vi "MultiScanDrift_v2.vi"() -> ()   [LabVIEW 2014]
uses:
  shared/CorrelImages (SubVI)Single.vi
  <userlib>/Nanonis Prog Interface V5/Nanonis Prog Interface.lvlib
panel:
  out "Direction: up/down (T=up)":bool
  in  "PLL ON/OFF":bool
  in  "ref bias":dbl=-0.0012 format="%#_6p"
  in  "ref setpoint":bool=TRUE
  in  "DC On":bool
  out "Y drift":i32
  out "X drift":i32
  out "DC active":bool
  in  "Drift correction Pixels":i32=256
  in  "Img Current":sgl=2.5e-11 format="%#_6p"
  in  "Img Bias (V) DC":sgl=0.02 format="%_2p"
  in  "Forward Speed":sgl=5e-10 format="%#_6p"
  in  "Backward Speed":sgl=8e-08 format="%#_6p"
  in  "Img Speed":sgl=3e-08 format="%#_6p"
  in  "Channel index (0-23)":u8(ring) items=["Current"=0, "Z (m)"=14]
  in  "Settling time (s)":dbl=0.7 format="%#_6p"
  in  "img bias":bool=TRUE
  in  "img bias":dbl=-0.0012 format="%#_6p"
  in  "img delay (s)":u32=1
  out "tipLift":dbl=1e-10 format="%#_6p"
  in  "TipLiftList":i32(listbox)
  in  "Const Height":bool=TRUE
  in  "CurrentList":i32(listbox)
  in  "BiasList":i32(listbox)
  out "Current":dbl=2.5e-11 format="%#_6p"
  out "Bias":dbl=0.02 format="%#_6p"
  # "Turn continuous scan off\n zero tiplift is '0'"
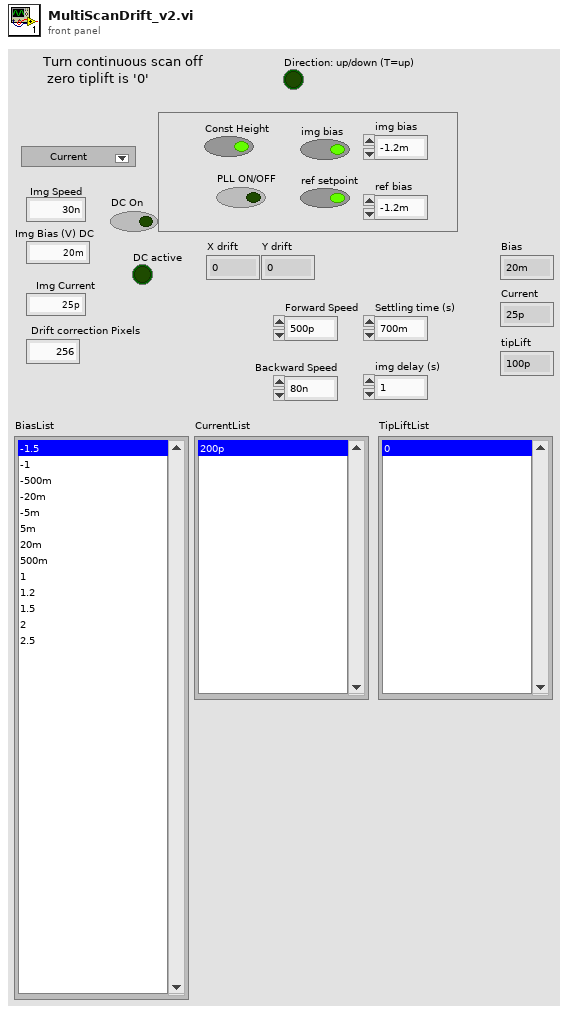
[diagram p1: front panel]
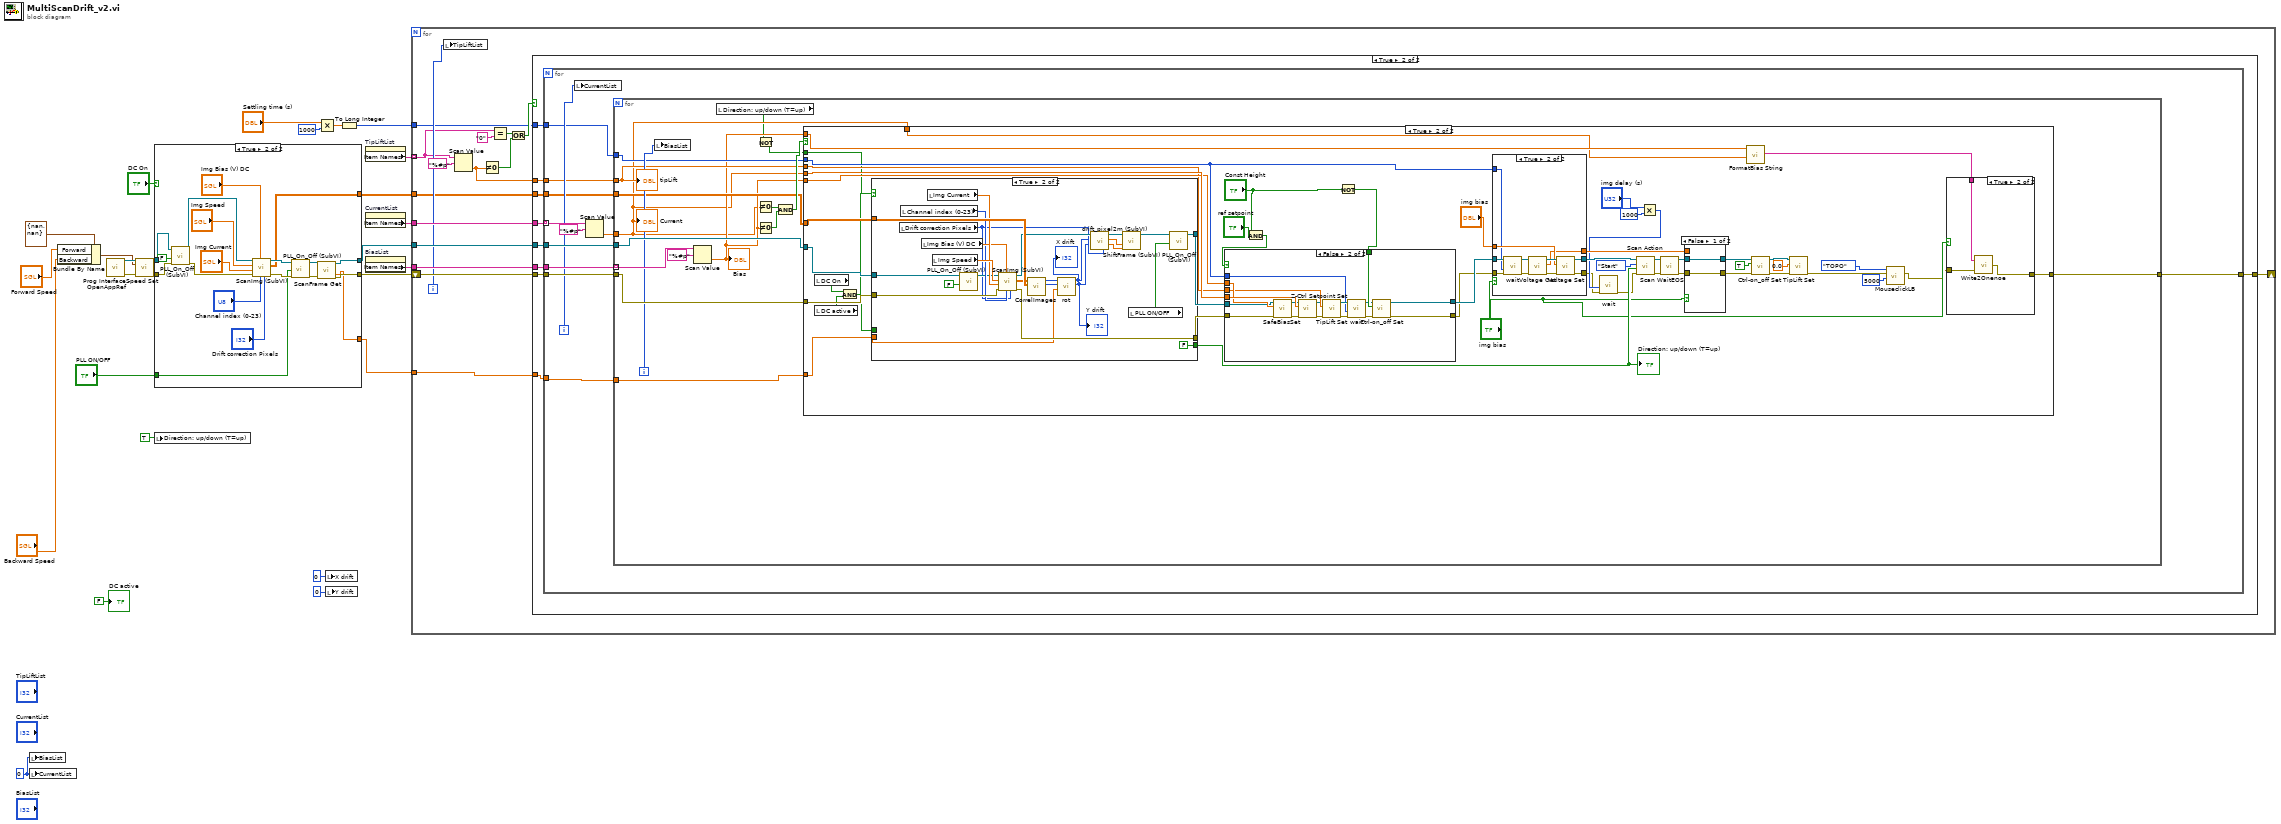
[diagram p0: block diagram]
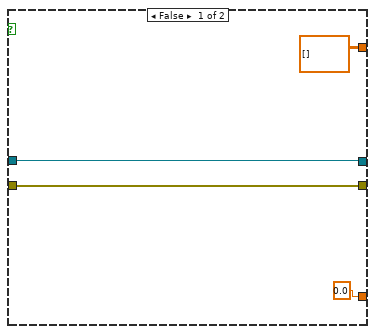
[diagram p2: hidden frame]
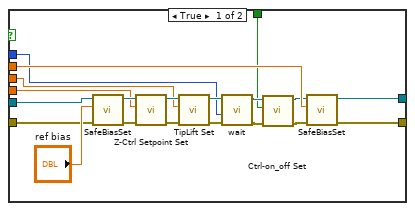
[diagram p5: hidden frame]
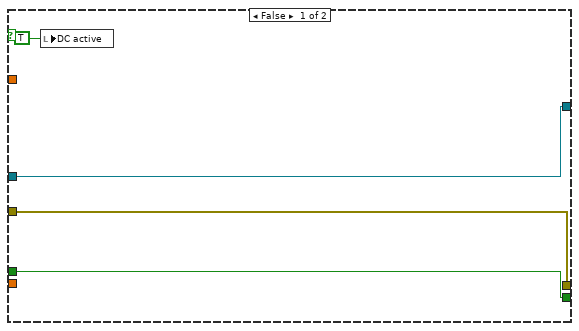
[diagram p7: hidden frame]
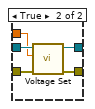
[diagram p8: hidden frame]
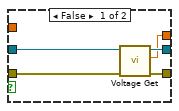
[diagram p9: hidden frame]
diagram:
  w26 = 0 ("BiasList")
  n1 = local write "BiasList"(w26) -> ()
  n2 = local write "CurrentList"(w26) -> ()
  n3 = Bundle By Name(cluster=cluster{"Forward":sgl, "Backward":sgl} {"Forward"=nan, "Backward"=nan} ("Speed (m/s)"), "Forward"="Forward Speed", "Backward"="Backward Speed") -> (w11:cluster{"Forward":sgl, "Backward":sgl})
  n4 = call <userlib>:"Prog Interface - OpenAppRef.vi"() -> ("Error out"=w12:errorcluster, "Application reference"=w13:refnum<vi>)  [unwired: 6 in]
  n5 = call <userlib>:"Speed Set.vi"("Application ref in"=w13, "Speed (m/s)"=w11, "error in (no error)"=w12) -> ("Application ref out"=w9:refnum<vi>, "error out"=w8:errorcluster)  [unwired: 11 in]
  n6 = case shown="True" "DC On" {
    tunnel: [w29 w34] -> w15
    tunnel: [w28 w33] -> w14
    tunnel: [dbl[][] [] ("Img") w43] -> w10
    tunnel: w9 -> [w29 w42]
    tunnel: w8 -> [w28 w40]
    tunnel: [sgl 0.0 ("Angle (deg)") w32] -> w3
    tunnel: "PLL ON/OFF" -> [_ w31]
    frame False {
    }
    frame True {
      n7 = call "PLL_On_Off (SubVI).vi"("error in (no error)"=w40, "Output ON/OFF (F=OFF)"=FALSE, "Application in"=w42) -> ("error out"=w39:errorcluster, "Application out"=w41:refnum<vi>)  [unwired: 7 in]
      n8 = call "ScanImg (SubVI).vi"("pixel"="Drift correction Pixels", "Channel index (0-23)"="Channel index (0-23)", "Bias (V)"="Img Bias (V) DC", "error in (no error)"=w39, "Current"="Img Current", "Img Speed"="Img Speed", "Application in"=w41) -> ("error out"=w46:errorcluster, "Img"=w43:dbl[][], "Application out"=w47:refnum<vi>)  [unwired: 2 in]
      n9 = call "PLL_On_Off (SubVI).vi"("error in (no error)"=w46, "Output ON/OFF (F=OFF)"=w31, "Application in"=w47) -> ("error out"=w35:errorcluster, "Application out"=w36:refnum<vi>)  [unwired: 7 in]
      n10 = call <userlib>:"ScanFrame Get.vi"("Application ref in"=w36, "error in (no error)"=w35) -> ("Application ref out"=w34:refnum<vi>, "Angle (deg)"=w32:sgl, "error out"=w33:errorcluster)  [unwired: 9 in, 2 out]
    }
  }
  n11 = local write "Direction: up/down (T=up)"(TRUE ("Direction: up/down (T=up)")) -> ()
  n12 = Multiply(x="Settling time (s)", y=u32 1000) -> (x*y=w22:dbl)
  n13 = local write "X drift"(0 ("X drift")) -> ()
  n14 = local write "Y drift"(0 ("Y drift")) -> ()
  n15 = To Long Integer(number=w22) -> (32bit integer=w23:i32)
  n16 = property on="TipLiftList" class="LstBox (strict)"() -> ("Item Names"=w19:string[])  [unwired: 2 in, 2 out]
  n17 = property on="CurrentList" class="LstBox (strict)"() -> ("Item Names"=w20:string[])  [unwired: 2 in, 2 out]
  n18 = property on="BiasList" class="LstBox (strict)"() -> ("Item Names"=w21:string[])  [unwired: 2 in, 2 out]
  n19 = for {
    tunnel: w21 -> [w65]
    tunnel: w20 -> [w64]
    tunnel: w15 -> [w63]
    tunnel: w19 -> [w59] mode=indexing
    tunnel: w23 -> [w53]
    tunnel: w10 -> [w52]
    tunnel: w3 -> [w51]
    shift-right: [w50] -> _
    shift-left: w14 -> [w62]
    i -> [w60]
    n20 = local write "TipLiftList"(w60) -> ()
    n21 = Scan Value(string=w59, format string="%#p") -> (value=w58:dbl)  [unwired: 1 in, 1 out]
    n22 = Not Equal To 0?(x=w58) -> (x != 0?=w57:bool)
    n23 = Equal?(x=w59, y="0") -> (x = y?=w54:bool)
    n24 = Or(x=w54, y=w57) -> (x .or. y?=w56:bool)
    n25 = case shown="True" w56 {
      tunnel: w65 -> [_ w75]
      tunnel: w64 -> [_ w74]
      tunnel: w63 -> [_ w73]
      tunnel: w62 -> [w66 w72]
      tunnel: w58 -> [_ w71]
      tunnel: w53 -> [_ w70]
      tunnel: w52 -> [_ w69]
      tunnel: w51 -> [_ w68]
      tunnel: [w66 w67] -> w50
      frame False {
      }
      frame True {
        n26 = for {
          tunnel: w73 -> [w87]
          tunnel: w72 -> [w86]
          tunnel: w75 -> [w85]
          tunnel: w74 -> [w83] mode=indexing
          tunnel: w71 -> [w80]
          tunnel: w70 -> [w79]
          tunnel: w69 -> [w78]
          tunnel: w68 -> [w77]
          tunnel: [w76] -> w67
          i -> [w81]
          n27 = local write "CurrentList"(w81) -> ()
          n28 = Scan Value(string=w83, format string="%#p") -> (value=w82:dbl)  [unwired: 1 in, 1 out]
          n29 = for {
            tunnel: w85 -> [w101] mode=indexing
            tunnel: w87 -> [w103]
            tunnel: w86 -> [w102]
            tunnel: w82 -> [w91]
            tunnel: w80 -> [w96]
            tunnel: w79 -> [w95]
            tunnel: w78 -> [w94]
            tunnel: w77 -> [w93]
            tunnel: [w90] -> w76
            i -> [w97]
            n30 = local write "BiasList"(w97) -> ()
            n31 = Scan Value(string=w101, format string="%#p") -> (value=w92:dbl)  [unwired: 1 in, 1 out]
            "Bias" <- w92
            n32 = local read "Direction: up/down (T=up)"() -> (w89:bool)
            n33 = Not(x=w89) -> (.not. x?=w88:bool)
            n34 = Not Equal To 0?(x=w91) -> (x != 0?=w100:bool)
            n35 = Not Equal To 0?(x=w92) -> (x != 0?=w99:bool)
            n36 = Compound Arithmetic op=AND(w100, w99) -> (w98:bool)
            n37 = case shown="True" w98 {
              tunnel: w88 -> [_ w119]
              tunnel: w92 -> [_ w153]
              tunnel: w103 -> [_ w126]
              tunnel: w102 -> [w105 w125]
              tunnel: w91 -> [_ w154]
              tunnel: w96 -> [_ w147]
              tunnel: w95 -> [_ w128]
              tunnel: w94 -> [_ w127]
              tunnel: w93 -> [_ w117]
              tunnel: w92 -> [_ w116]
              tunnel: w91 -> [_ w115]
              tunnel: [w105 w112] -> w90
              frame False {
              }
              frame True {
                n38 = local read "DC On"() -> (w121:bool)
                n39 = local read "DC active"() -> (w122:bool)
                n40 = And(x=w121, y=w122) -> (x .and. y?=w120:bool)
                n41 = case shown="True" w120 {
                  tunnel: w127 -> [_ w224]
                  tunnel: w126 -> [w198 w212]
                  tunnel: w125 -> [w199 w223]
                  tunnel: [w199 w222] -> w124
                  tunnel: [w198 w209] -> w123
                  tunnel: [w196 FALSE ("Direction: up/down (T=up)")] -> w118
                  tunnel: w119 -> [w196 _]
                  tunnel: w117 -> [_ w205]
                  frame False {
                    n42 = local write "DC active"(TRUE ("DC active")) -> ()
                  }
                  frame True {
                    n43 = local read "Drift correction Pixels"() -> (w207:i32)
                    n44 = local read "Channel index (0-23)"() -> (w217:u8)
                    n45 = local read "Img Bias (V) DC"() -> (w218:sgl)
                    n46 = local read "Img Current"() -> (w219:sgl)
                    n47 = local read "Img Speed"() -> (w220:sgl)
                    n48 = call "PLL_On_Off (SubVI).vi"("Output ON/OFF (F=OFF)"=FALSE, "Application in"=w212) -> ("Application out"=w211:refnum<vi>)  [unwired: 8 in, 1 out]
                    n49 = call "ScanImg (SubVI).vi"("pixel"=w207, "Channel index (0-23)"=w217, "Bias (V)"=w218, "error in (no error)"=w223, "Current"=w219, "Img Speed"=w220, "Application in"=w211) -> ("error out"=w222:errorcluster, "Img"=w221:dbl[][], "Application out"=w213:refnum<vi>)  [unwired: 2 in]
                    n50 = call-poly "CorrelImages.vi"("Ref Array"=w224, "New Image"=w221) -> ("Y drift"=w202:i32, "X drift"=w204:i32)  [unwired: 6 in, 2 out]
                    n51 = call "rot.vi"("angle"=w205, "y"=w202, "x"=w204) -> ("y'"=w201:i32, "x'"=w203:i32)  [unwired: 7 in]
                    "X drift" <- w203
                    "Y drift" <- w201
                    n52 = call "drift_pixel2m (SubVI).vi"("Application in"=w213, "X drift"=w203, "Y drift"=w201, "Drift correction Pixels"=w207) -> ("Application out"=w214:refnum<vi>, "x drift"=w216:sgl, "y drift"=w215:sgl)  [unwired: 2 in, 1 out]
                    n53 = call "ShiftFrame (SubVI).vi"("Y shift"=w215, "X shift"=w216, "Application in"=w214) -> ("Application out"=w210:refnum<vi>)  [unwired: 8 in]
                    n54 = local read "PLL ON/OFF"() -> (w200:bool)
                    n55 = call "PLL_On_Off (SubVI).vi"("Output ON/OFF (F=OFF)"=w200, "Application in"=w210) -> ("Application out"=w209:refnum<vi>)  [unwired: 8 in, 1 out]
                  }
                }
                "Direction: up/down (T=up)" <- w118
                n56 = And(x="Const Height", y="ref setpoint") -> (x .and. y?=w109:bool)
                n57 = Not(x="Const Height") -> (.not. x?=w150:bool)
                n58 = case shown="False" w109 {
                  tunnel: w154 -> [w162 w191]
                  tunnel: w153 -> [w174 w190]
                  tunnel: w150 -> [w155 w189]
                  tunnel: w147 -> [w163 w187]
                  tunnel: [w157 w186] -> w144
                  tunnel: [w156 w185] -> w142
                  tunnel: w128 -> [w164 w181]
                  tunnel: w124 -> [w160 w180]
                  tunnel: w123 -> [w161 w179]
                  frame True {
                    n59 = call "SafeBiasSet.vi"("Application ref in"=w161, "Bias (V)"="ref bias", "error in (no error)"=w160) -> ("Application ref out"=w171:refnum<vi>, "Error out"=w173:errorcluster)  [unwired: 6 in]
                    n60 = call <userlib>:"Z-Ctrl Setpoint Set.vi"("error in (no error)"=w173, "Z Controller setpoint"=w162, "Application ref in"=w171) -> ("error out"=w166:errorcluster, "Application ref out"=w168:refnum<vi>)  [unwired: 7 in]
                    n61 = call <userlib>:"TipLift Set.vi"("error in (no error)"=w166, "TipLift (m)"=w163, "Application ref in"=w168) -> ("error out"=w165:errorcluster, "Application ref out"=w167:refnum<vi>)  [unwired: 7 in]
                    n62 = call "wait.vi"("error in"=w165, "milliseconds to wait"=w164, "application reference in"=w167) -> ("error out"=w170:errorcluster, "application reference out"=w169:refnum<vi>)  [unwired: 7 in]
                    n63 = call <userlib>:"Ctrl-on_off Set.vi"("error in (no error)"=w170, "Z Controller ON/OFF"=w155, "Application ref in"=w169) -> ("error out"=w158:errorcluster, "Application ref out"=w159:refnum<vi>)  [unwired: 7 in]
                    n64 = call "SafeBiasSet.vi"("Application ref in"=w159, "Bias (V)"=w174, "error in (no error)"=w158) -> ("Application ref out"=w157:refnum<vi>, "Error out"=w156:errorcluster)  [unwired: 6 in]
                  }
                  frame False {
                    n65 = call "SafeBiasSet.vi"("Application ref in"=w179, "Bias (V)"=w190, "error in (no error)"=w180) -> ("Application ref out"=w178:refnum<vi>, "Error out"=w177:errorcluster)  [unwired: 6 in]
                    n66 = call <userlib>:"Z-Ctrl Setpoint Set.vi"("error in (no error)"=w177, "Z Controller setpoint"=w191, "Application ref in"=w178) -> ("error out"=w175:errorcluster, "Application ref out"=w176:refnum<vi>)  [unwired: 7 in]
                    n67 = call <userlib>:"TipLift Set.vi"("error in (no error)"=w175, "TipLift (m)"=w187, "Application ref in"=w176) -> ("error out"=w182:errorcluster, "Application ref out"=w188:refnum<vi>)  [unwired: 7 in]
                    n68 = call "wait.vi"("error in"=w182, "milliseconds to wait"=w181, "application reference in"=w188) -> ("error out"=w183:errorcluster, "application reference out"=w184:refnum<vi>)  [unwired: 7 in]
                    n69 = call <userlib>:"Ctrl-on_off Set.vi"("error in (no error)"=w183, "Z Controller ON/OFF"=w189, "Application ref in"=w184) -> ("error out"=w185:errorcluster, "Application ref out"=w186:refnum<vi>)  [unwired: 7 in]
                  }
                }
                n70 = case shown="True" "img bias" {
                  tunnel: w144 -> [w236 w238]
                  tunnel: [w235 w245] -> w143
                  tunnel: w142 -> [w232 w241]
                  tunnel: [w233 w244] -> w107
                  tunnel: "img bias" -> [_ w243]
                  tunnel: [w234 w242] -> w140
                  tunnel: w128 -> [_ w237]
                  frame False {
                    n71 = call <userlib>:"Voltage Get.vi"("error in (no error)"=w232, "Application ref in"=w236) -> ("error out"=w233:errorcluster, "Bias (V)"=w234:sgl, "Application ref out"=w235:refnum<vi>)  [unwired: 7 in]
                  }
                  frame True {
                    n72 = call "wait.vi"("error in"=w241, "milliseconds to wait"=w237, "application reference in"=w238) -> ("error out"=w240:errorcluster, "application reference out"=w239:refnum<vi>)  [unwired: 7 in]
                    n73 = call <userlib>:"Voltage Get.vi"("error in (no error)"=w240, "Application ref in"=w239) -> ("error out"=w247:errorcluster, "Bias (V)"=w242:sgl, "Application ref out"=w246:refnum<vi>)  [unwired: 7 in]
                    n74 = call <userlib>:"Voltage Set.vi"("Error in (no error)"=w247, "Bias (V)"=w243, "Application ref in"=w246) -> ("Error out"=w244:errorcluster, "Application ref out"=w245:refnum<vi>)  [unwired: 7 in]
                  }
                }
                n75 = Multiply(x="img delay (s)", y=u32 1000) -> (x*y=w129:u32)
                n76 = call "wait.vi"("error in"=w107, "milliseconds to wait"=w129) -> ("error out"=w106:errorcluster)  [unwired: 8 in, 1 out]
                n77 = call <userlib>:"Scan Action.vi"("error in (no error)"=w106, "Direction: up/down (T=up)"=w118, "Scan action (Start)"=enum16{"Start", "Stop", "Pause", "Resume"}."Start", "Application ref in"=w143) -> ("error out"=w152:errorcluster, "Application ref out"=w151:refnum<vi>)  [unwired: 5 in]
                n78 = call <userlib>:"Scan WaitEOS.vi"("error in (no error)"=w152, "Application ref in"=w151) -> ("error out"=w138:errorcluster, "Application ref out"=w139:refnum<vi>)  [unwired: 5 in, 2 out]
                n79 = case shown="False" "img bias" {
                  tunnel: w139 -> [w226 w229]
                  tunnel: [w226 w231] -> w137
                  tunnel: [w225 w230] -> w136
                  tunnel: w138 -> [w225 w228]
                  tunnel: w140 -> [_ w227]
                  frame False {
                  }
                  frame True {
                    n80 = call <userlib>:"Voltage Set.vi"("Error in (no error)"=w228, "Bias (V)"=w227, "Application ref in"=w229) -> ("Error out"=w230:errorcluster, "Application ref out"=w231:refnum<vi>)  [unwired: 7 in]
                  }
                }
                n81 = call "FormatBias String.vi"("current"=w115, "bias"=w116) -> ("resulting string"=w113:string)  [unwired: 9 in]
                n82 = call <userlib>:"Ctrl-on_off Set.vi"("error in (no error)"=w136, "Z Controller ON/OFF"=TRUE, "Application ref in"=w137) -> ("error out"=w135:errorcluster, "Application ref out"=w134:refnum<vi>)  [unwired: 7 in]
                n83 = call <userlib>:"TipLift Set.vi"("error in (no error)"=w135, "TipLift (m)"=sgl 0.0, "Application ref in"=w134) -> ("error out"=w146:errorcluster)  [unwired: 7 in, 1 out]
                n84 = call "MouseclickLB.vi"("nMilliseconds"=5000, "error in (no error)"=w146, "Click"=enum16{"Header", "TOPO", "STS", "GRID"}."TOPO") -> ("error out"=w108:errorcluster)  [unwired: 8 in]
                n85 = case shown="True" "img bias" {
                  tunnel: w108 -> [w192 w195]
                  tunnel: w113 -> [_ w194]
                  tunnel: [w192 w193] -> w112
                  frame False {
                  }
                  frame True {
                    n86 = call "Write2Onenoe.vi"("error in (no error)"=w195, "strSendText"=w194) -> ("error out"=w193:errorcluster)
                  }
                }
              }
            }
            "Current" <- w91
            "tipLift" <- w96
          }
        }
      }
    }
  }
  "DC active" <- FALSE ("DC active")
